vi "String to Tag.vi"(9 "byte order":T1(ring), 10 "file refnum":refnum<file>, 11 "Binary Tag String":string) -> (2 "refnum out":refnum<file>, 3 "Tag Array":refnum<class "IFD_Tag.lvclass">[](array[class]))   [LabVIEW 2016]
uses:
  Class/Tag/IFD_Tag.lvclass
  Class/Tag/IFD_Tag.lvclass/IFD_Tag.ctl
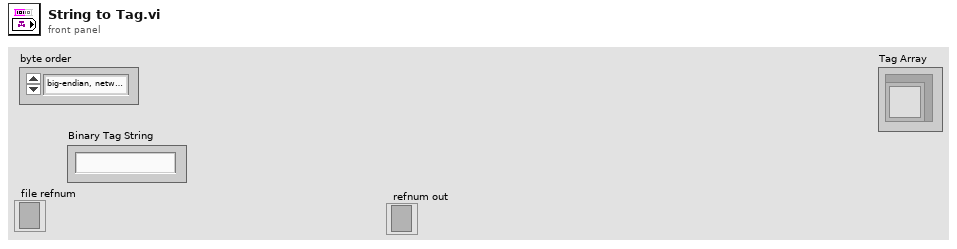
[diagram p1: front panel]
types:
  T1 = enum16{"big-endian, network order", "native, host order", "little-endian"}
  T2 = cluster{"Tag ID":u16, "Data Type":enum16{"Undefined(DO NOT USE)", "U8", "ASCII", "U16", "U32", "RATIONAL", "I8", "Undefined 8 bit", "I16", "I32", "SRATIONAL", "SGL", "DBL"}, "Data Count":u32}
  T3 = enum16{"Undefined(DO NOT USE)", "U8", "ASCII", "U16", "U32", "RATIONAL", "I8", "Undefined 8 bit", "I16", "I32", "SRATIONAL", "SGL", "DBL"}
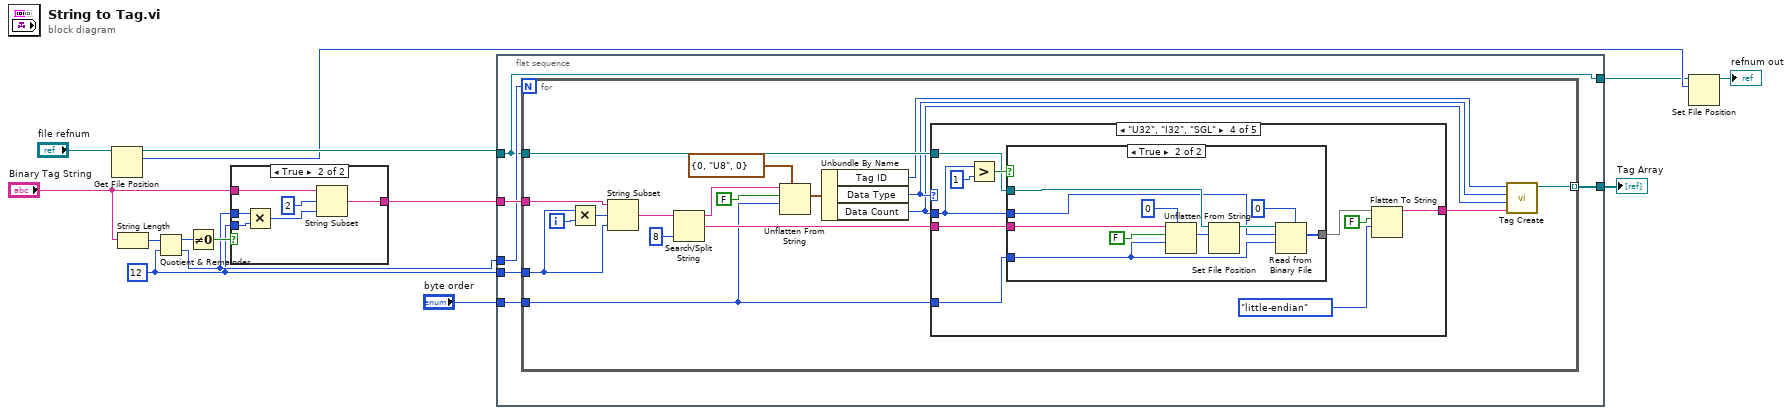
[diagram p0: block diagram]
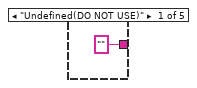
[diagram p2: hidden frame]
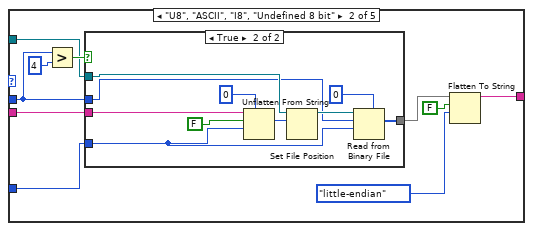
[diagram p3: hidden frame]
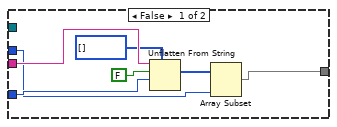
[diagram p4: hidden frame]
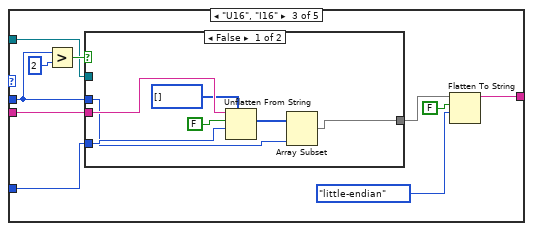
[diagram p5: hidden frame]
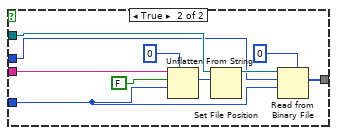
[diagram p6: hidden frame]
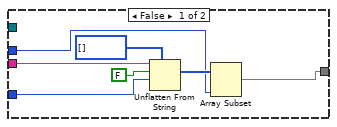
[diagram p7: hidden frame]
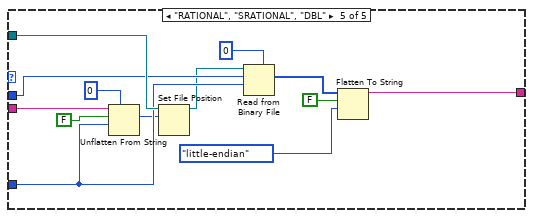
[diagram p8: hidden frame]
diagram:
  w8 = 12 ("y")
  n1 = Get File Position(7:"file refnum") -> (2:w4:i64, 3:w5:refnum<file>)  [unwired: 1 in, 1 out]
  n2 = String Length(string="Binary Tag String") -> (length=w14:i32)
  n3 = Quotient & Remainder(x=w14, y=w8) -> (x-y*floor(x/y)=w13:i32, floor(x/y)=w9:i32)
  n4 = Not Equal To 0?(x=w13) -> (x != 0?=w12:bool)
  n5 = case shown="True" w12 {
    tunnel: w9 -> [_ w21]
    tunnel: w8 -> [_ w20]
    tunnel: "Binary Tag String" -> [w15 w19]
    tunnel: [w15 w16] -> w10
    frame False {
    }
    frame True {
      n6 = Multiply(x=w21, y=w20) -> (x*y=w17:i32)
      n7 = String Subset(string=w19, offset (0)=2, length (rest)=w17) -> (substring=w16:string)
    }
  }
  n8 = flat-sequence {
    tunnel: w10 -> [w27]
    tunnel: w9 -> [w26]
    tunnel: w8 -> [w25]
    tunnel: "byte order" -> [w24]
    tunnel: w5 -> [w23]
    tunnel: [w23] -> w2
    tunnel: [w22] -> w1
    frame #0 {
      n9 = for {
        N: w26 -> [_]
        tunnel: w27 -> [w45]
        tunnel: w25 -> [w42]
        tunnel: w24 -> [w33]
        tunnel: w23 -> [w34]
        tunnel: [w28] -> w22 mode=indexing
        i -> [w44]
        n10 = Multiply(x=w42, y=w44) -> (x*y=w43:i32)
        n11 = String Subset(string=w45, offset (0)=w43, length (rest)=w42) -> (substring=w41:string)
        n12 = Search/Split String(string=w41, offset (0)=8) -> (substring before match=w39:string, match + rest of string=w35:string)  [unwired: 1 in, 1 out]
        n13 = Unflatten From String(type=T2 {"Tag ID"=0, "Data Type"=enum."U8", "Data Count"=0}, binary string=w39, data includes array or string size? (T)=FALSE, byte order (0:big-endian, network order)=w33) -> (value=w36:T2)  [unwired: 1 in, 2 out]
        n14 = Unbundle By Name(w36) -> ("Tag ID"=w32:u16, "Data Type"=w31:T3, "Data Count"=w30:u32)
        n15 = case shown="\"U32\", \"I32\", \"SGL\"" w31 {
          tunnel: w35 -> [_ w53 w80 w107 w139]
          tunnel: ["" w50 w77 w104 w136] -> w29
          tunnel: w30 -> [_ w52 w79 w106 w138]
          tunnel: w34 -> [_ w54 w81 w108 w140]
          tunnel: w33 -> [_ w49 w76 w103 w135]
          frame "Undefined(DO NOT USE)" {
          }
          frame "U8", "ASCII", "I8", "Undefined 8 bit" {
            n16 = Greater?(x=w52, y=u32 4) -> (0:w55:bool)
            n17 = case shown="True" w55 {
              tunnel: w54 -> [_ w70]
              tunnel: w53 -> [w63 w73]
              tunnel: w49 -> [w62 w65]
              tunnel: w52 -> [w57 w67]
              tunnel: [w58 w64] -> w48
              frame False {
                n18 = Unflatten From String(type=u8[] [], binary string=w63, data includes array or string size? (T)=FALSE, byte order (0:big-endian, network order)=w62) -> (value=w60:u8[])  [unwired: 1 in, 2 out]
                n19 = Array Subset(array=w60, length=w57) -> (w58:u8[])  [unwired: 1 in]
              }
              frame True {
                n20 = Unflatten From String(type=u32 0, binary string=w73, data includes array or string size? (T)=FALSE, byte order (0:big-endian, network order)=w65) -> (value=w69:u32)  [unwired: 1 in, 2 out]
                n21 = Set File Position(offset (in bytes) (0)=w69, refnum=w70) -> (refnum out=w68:refnum<file>)  [unwired: 2 in, 1 out]
                n22 = Read from Binary File(5:u8 0, 9:w65, 10:w67, 11:w68) -> (2:w64:u8[])  [unwired: 2 in, 3 out]
              }
            }
            n23 = Flatten To String(anything=w48, prepend array or string size? (T)=FALSE, byte order (0:big-endian, network order)=T1."little-endian") -> (data string=w50:string)  [unwired: 1 in, 2 out]
          }
          frame "U16", "I16" {
            n24 = Greater?(x=w79, y=u32 2) -> (0:w82:bool)
            n25 = case shown="False" w82 {
              tunnel: w81 -> [_ w97]
              tunnel: w80 -> [w90 w100]
              tunnel: w76 -> [w89 w92]
              tunnel: w79 -> [w84 w94]
              tunnel: [w85 w91] -> w75
              frame False {
                n26 = Unflatten From String(type=u16[] [], binary string=w90, data includes array or string size? (T)=FALSE, byte order (0:big-endian, network order)=w89) -> (value=w87:u16[])  [unwired: 1 in, 2 out]
                n27 = Array Subset(array=w87, length=w84) -> (w85:u16[])  [unwired: 1 in]
              }
              frame True {
                n28 = Unflatten From String(type=u32 0, binary string=w100, data includes array or string size? (T)=FALSE, byte order (0:big-endian, network order)=w92) -> (value=w96:u32)  [unwired: 1 in, 2 out]
                n29 = Set File Position(offset (in bytes) (0)=w96, refnum=w97) -> (refnum out=w95:refnum<file>)  [unwired: 2 in, 1 out]
                n30 = Read from Binary File(5:u16 0, 9:w92, 10:w94, 11:w95) -> (2:w91:u16[])  [unwired: 2 in, 3 out]
              }
            }
            n31 = Flatten To String(anything=w75, prepend array or string size? (T)=FALSE, byte order (0:big-endian, network order)=T1."little-endian") -> (data string=w77:string)  [unwired: 1 in, 2 out]
          }
          frame "U32", "I32", "SGL" {
            n32 = Greater?(x=w106, y=u32 1) -> (0:w109:bool)
            n33 = case shown="True" w109 {
              tunnel: w108 -> [_ w124]
              tunnel: w107 -> [w117 w127]
              tunnel: w103 -> [w116 w119]
              tunnel: w106 -> [w111 w121]
              tunnel: [w112 w118] -> w102
              frame False {
                n34 = Unflatten From String(type=u32[] [], binary string=w117, data includes array or string size? (T)=FALSE, byte order (0:big-endian, network order)=w116) -> (value=w114:u32[])  [unwired: 1 in, 2 out]
                n35 = Array Subset(array=w114, length=w111) -> (w112:u32[])  [unwired: 1 in]
              }
              frame True {
                n36 = Unflatten From String(type=u32 0, binary string=w127, data includes array or string size? (T)=FALSE, byte order (0:big-endian, network order)=w119) -> (value=w123:u32)  [unwired: 1 in, 2 out]
                n37 = Set File Position(offset (in bytes) (0)=w123, refnum=w124) -> (refnum out=w122:refnum<file>)  [unwired: 2 in, 1 out]
                n38 = Read from Binary File(5:u32 0, 9:w119, 10:w121, 11:w122) -> (2:w118:u32[])  [unwired: 2 in, 3 out]
              }
            }
            n39 = Flatten To String(anything=w102, prepend array or string size? (T)=FALSE, byte order (0:big-endian, network order)=T1."little-endian") -> (data string=w104:string)  [unwired: 1 in, 2 out]
          }
          frame "RATIONAL", "SRATIONAL", "DBL" {
            n40 = Unflatten From String(type=u32 0, binary string=w139, data includes array or string size? (T)=FALSE, byte order (0:big-endian, network order)=w135) -> (value=w131:u32)  [unwired: 1 in, 2 out]
            n41 = Set File Position(offset (in bytes) (0)=w131, refnum=w140) -> (refnum out=w130:refnum<file>)  [unwired: 2 in, 1 out]
            n42 = Read from Binary File(5:u64 0, 9:w135, 10:w138, 11:w130) -> (2:w134:u64[])  [unwired: 2 in, 3 out]
            n43 = Flatten To String(anything=w134, prepend array or string size? (T)=FALSE, byte order (0:big-endian, network order)=T1."little-endian") -> (data string=w136:string)  [unwired: 1 in, 2 out]
          }
        }
        n44 = call "Tag Create.vi"("Data"=w29, "Data Count"=w30, "Data Type"=w31, "Tag ID"=w32) -> ("IFD_Tag out"=w28:refnum<class "IFD_Tag.lvclass">)  [unwired: 7 in]
      }
    }
  }
  n45 = Set File Position(offset (in bytes) (0)=w4, refnum=w2) -> (refnum out=→"refnum out":refnum<file>)  [unwired: 2 in, 1 out]
  "Tag Array" <- w1
